vi "XIPIN_CIC_Compiler_2_0.vi"   [LabVIEW 2017]
doc: "The Xilinx CIC Compiler LogiCORE is a module for design and implementation of Cascaded Integrator-Comb (CIC) filters for a variety of Xilinx FPGA devices\n------------------------------------\n<b>Need License</b> : No"
uses:
  <vilib>/rvi/XilinxIP/XIPIN_XNode/niFpgaXIPIN.xnode
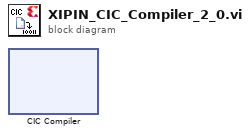
[diagram p0: block diagram]
diagram:
  n1 = xnode ("CIC Compiler")() -> ()
